vi "高亮显示单击的行.vi"() -> ()   [LabVIEW 2013, in "Table Tool.lvlib"]
uses:
  Table Tool.lvlib
  Custum Type/Selet Row or Col.ctl
  Custum Type/GetOrSet.ctl
  Property/Set Or get Row Head and Column Head Strings.vi
panel:
  in  "Headers[] In":string[](array[string])=["##", "####", "#####", "#########", "############"]
  in  "停止":bool
  in  "Origin BK Color":u32(colorbox)=16448250
  in  "BK Color In":u32(colorbox)=13816530
  out "Highlight Clicked Row":string[][](table)=[["%%", "", "", "", ""], ["", "%%%", "", "", ""], ["", "", "%%%", "", ""], ["", "", "", "", ""], ["", "", "", "%%%%", ""], ["", "", "", "", ""], ["", "", "", "", ""], ["", "", "", "", ""], ["", "", "", "", ""], ["", "", "", "", ""], ["", "", "", "", "%%%%"]]
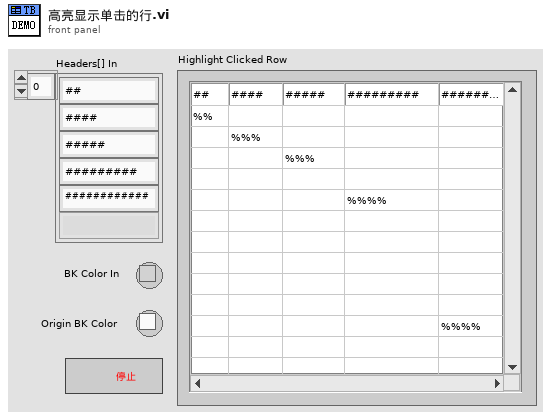
[diagram p1: front panel]
types:
  T1 = typedef "Table Tool.lvlib/GetOrSet.ctl" = enum16{"Get", "Set"}
  T2 = typedef "Table Tool.lvlib/Selet Row or Col.ctl" = enum16{"Col", "Row"}
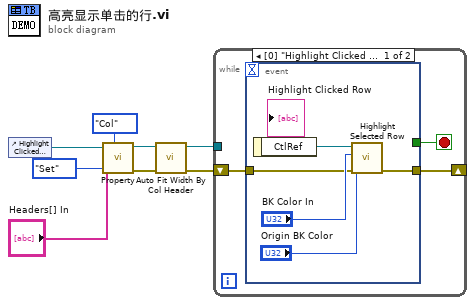
[diagram p0: block diagram]
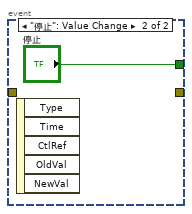
[diagram p2: hidden frame]
diagram:
  n1 = control-ref of="Highlight Clicked Row"() -> (w7:refnum<vi>)
  n2 = call-poly "Property.vi"("Row or Col Option"=Selet_Row_or_Col."Col", "Mode"=GetOrSet."Set", "Headers[] In"="Headers[] In", "Table Ref In"=w7) -> ("error out"=w3:errorcluster, "Table Ref Out"=w4:refnum<vi>)  [unwired: 5 in, 1 out]
  n3 = call "Auto Fit Width By Col Header.vi"("error in (no error)"=w3, "Table Ref In"=w4) -> ("error out"=w2:errorcluster, "Table Ref Out"=w1:refnum<vi>)  [unwired: 8 in]
  n4 = while {
    shift-right: [w9] -> _
    shift-left: w2 -> [w10]
    tunnel: w1 -> [_]
    stop <- w11 stop-if-true
    n5 = event shown="[0] \"Highlight Clicked Row\": 鼠标按下" {
      selector: _ -> [_ _]
      dyn-events: _ -> [_ _]
      timeout: _ -> [_ _]
      tunnel: [_ "停止"] -> w11
      tunnel: w10 -> [w13 _]
      tunnel: [w12 _] -> w9
      event "Highlight Clicked Row": Mouse Down {
        n6 = event-data() -> ("CtlRef"=w14:refnum<vi>)  [unwired: 1 in]
        n7 = call "Highlight Selected Row.vi"("error in (no error)"=w13, "Origin BK Color"="Origin BK Color", "BK Color In"="BK Color In", "Table Ref In"=w14) -> ("error out"=w12:errorcluster)  [unwired: 6 in, 1 out]
      }
      event "停止": Value Change {
        n8 = event-data() -> ()  [unwired: 1 in, 5 out]
      }
    }
  }
